vi "Initialize.vi"(7 "Baud Rate":u32(ring)=19200 items=["4800"=4800, "9600"=9600, "14400"=14400, "19200"=19200, "38400"=38400, "57600"=57600, "115200"=115200], 8 "error in (no error)":errorcluster, 9 "Reset (True)":bool=TRUE, 10 "ID Query (False)":bool, 11 "VISA resource name":refnum<visa-resource-name>) -> (0 "error out":errorcluster, 3 "VISA resource name out":refnum<visa-resource-name>)   [LabVIEW 2011, in "Ocean Server OS4000.lvlib"]
doc: "Establishes communication with the instrument and performs an instrument identification query. It also places the instrument in a default state needed for other instrument driver operations. Therefore, call this VI before calling other instrument driver VIs for this instrument. Generally, you need to call the Initialize VI only once at the beginning of an application."
uses:
  Ocean Server OS4000.lvlib
panel:
  # "(c) 2006 <National Instruments>.  ALL RIGHTS RESERVED."
  # "(c) 2009 National Instruments.  ALL RIGHTS RESERVED."
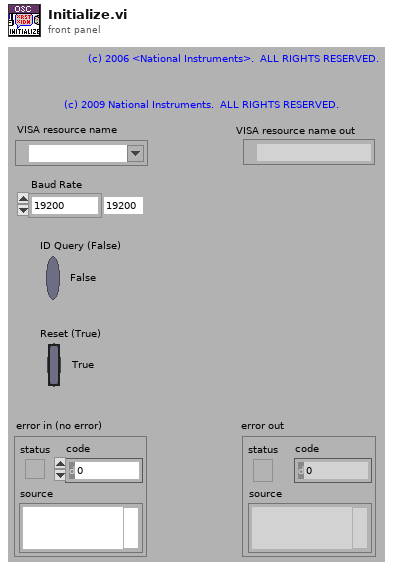
[diagram p1: front panel]
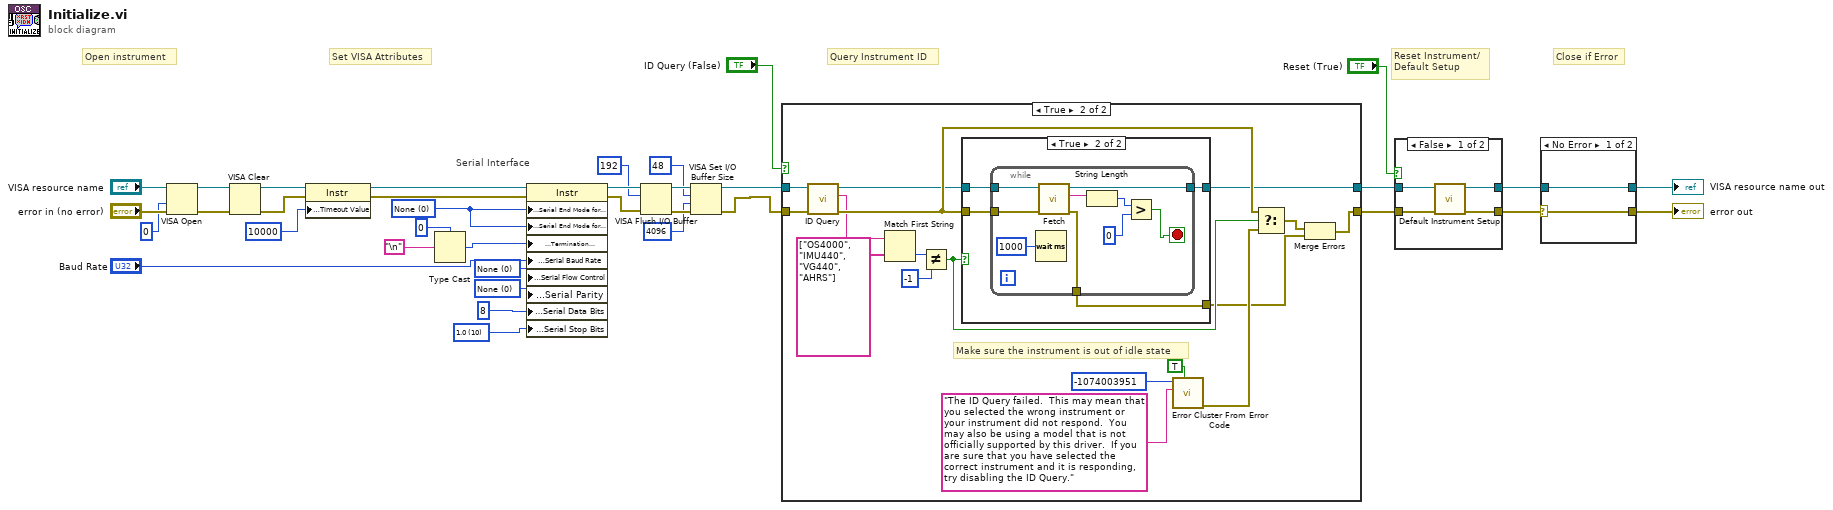
[diagram p0: block diagram]
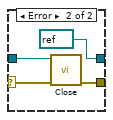
[diagram p2: hidden frame]
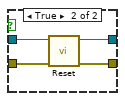
[diagram p3: hidden frame]
diagram:
  w1 = u16 10 items=["1.0"=10, "1.5"=15, "2.0"=20] ("Serial Settings:Stop Bits")
  w3 = u16 0 items=["None", "Odd", "Even", "Mark", "Space"] ("Serial Settings:Parity")
  w4 = u16 0 items=["None", "XON/XOFF", "RTS/CTS", "XON/XOFF & RTS/CTS", "DTR/DSR", "XON/XOFF & DTR/DSR"] ("Serial Settings:Flow Control")
  w8 = u16 0 items=["None", "LastBit", "TermChar"] ("Serial Settings:Serial End Mode for Reads")
  # "Serial Interface"
  # "Set VISA Attributes"
  # "Close if Error"
  # "Query Instrument ID"
  # "Reset Instrument/\nDefault Setup"
  # "Open instrument"
  n1 = VISA Open(access mode=u32 0, error in (no error)="error in (no error)", VISA resource name="VISA resource name") -> (VISA resource name=w24:refnum<visa-resource-name>, error out=w23:errorcluster)  [unwired: 2 in]
  n2 = VISA Clear(VISA resource name=w24, error in (no error)=w23) -> (VISA resource name out=w22:refnum<visa-resource-name>, error out=w21:errorcluster)
  n3 = property on="Property Node" class="Instr"(reference=w22, error in=w21, "General Settings:Timeout Value"=u32 10000) -> (reference out=w27:refnum<visa-resource-name>, error out=w26:errorcluster)
  n4 = Type Cast(type=0, x="\n" ("Line Feed Constant")) -> (*(type *) &x=w5:i32)
  n5 = property on="Property Node" class="Instr"(reference=w27, error in=w26, "Serial Settings:Serial End Mode for Reads"=w8, "Serial Settings:Serial End Mode for Writes"=w8, "Message Based Settings:Termination Character"=w5, "Serial Settings:Serial Baud Rate"="Baud Rate", "Serial Settings:Serial Flow Control"=w4, "Serial Settings:Serial Parity"=w3, "Serial Settings:Serial Data Bits"=u16 8 ("Serial Settings:Data Bits"), "Serial Settings:Serial Stop Bits"=w1) -> (reference out=w12:refnum<visa-resource-name>, error out=w14:errorcluster)
  n6 = VISA Flush I/O Buffer(VISA resource name=w12, mask (16)=u16 192, error in (no error)=w14) -> (VISA resource name out=w15:refnum<visa-resource-name>, error out=w13:errorcluster)
  n7 = VISA Set I/O Buffer Size(VISA resource name=w15, mask (16)=u16 48, size (4096)=u32 4096 ("size (0)"), error in (no error)=w13) -> (VISA resource name out=w29:refnum<visa-resource-name>, error out=w28:errorcluster)
  n8 = case shown="True" "ID Query (False)" {
    tunnel: [w37 w40] -> w35
    tunnel: [w38 w43] -> w36
    tunnel: w29 -> [w38 w51]
    tunnel: w28 -> [w37 w50]
    frame False {
    }
    frame True {
      # "Make sure the instrument is out of idle state"
      n9 = call "ID Query.vi"("error in (no error)"=w50, "VISA resource name"=w51) -> ("error out"=w45:errorcluster, "Model Name"=w39:string, "VISA resource name out"=w44:refnum<visa-resource-name>)  [unwired: 6 in, 1 out]
      n10 = Match First String(2:string[] ["OS4000", "IMU440", "VG440", "AHRS"], 3:w39) -> (0:w48:i32)  [unwired: 1 out]
      n11 = Not Equal?(x=w48, y=-1) -> (x != y?=w46:bool)
      n12 = case shown="True" w46 {
        tunnel: w44 -> [w57 w61]
        tunnel: w45 -> [w56 w60]
        tunnel: [w57 w59] -> w43
        tunnel: [w56 w58] -> w42
        frame False {
        }
        frame True {
          n13 = while {
            tunnel: w61 -> [w70]
            tunnel: w60 -> [w65]
            tunnel: [w64] -> w59
            tunnel: [w63] -> w58
            stop <- w66 stop-if-true
            n14 = Wait (ms)(milliseconds to wait=u32 1000) -> ()  [unwired: 1 out]
            n15 = call "Fetch.vi"("error in (no error)"=w65, "VISA resource name"=w70) -> ("error out"=w63:errorcluster, "Read Buffer"=w69:string, "VISA resource name out"=w64:refnum<visa-resource-name>)  [unwired: 5 in]
            n16 = String Length(string=w69) -> (length=w68:i32)
            n17 = Greater?(x=w68, y=0) -> (0:w66:bool)
          }
        }
      }
      n18 = call <vilib>:"Error Cluster From Error Code.vi"("show call chain? (False)"=TRUE, "error message (\"\")"="The ID Query failed.  This may mean that you selected the wrong instrument or your instrument did not respond.  You may also be using a model that is not officially supported by this driver.  If you are sure that you have selected the correct instrument and it is responding, try disabling the ID Query." ("Source (VI Name)"), "error code (0)"=-1074003951 ("Code")) -> ("error out"=w55:errorcluster)  [unwired: 6 in]
      n19 = Select(t=w45, s=w46, f=w55) -> (s? t:f=w41:errorcluster)
      n20 = Merge Errors(w41, w42) -> (w40:errorcluster)
    }
  }
  n21 = case shown="False" "Reset (True)" {
    tunnel: w35 -> [w73 w77]
    tunnel: [w71 w75] -> w17
    tunnel: w36 -> [w74 w78]
    tunnel: [w72 w76] -> w18
    frame False {
      n22 = call "Default Instrument Setup.vi"("error in (no error)"=w73, "VISA resource name"=w74) -> ("error out"=w71:errorcluster, "VISA resource out"=w72:refnum<visa-resource-name>)  [unwired: 8 in]
    }
    frame True {
      n23 = call "Reset.vi"("error in (no error)"=w77, "VISA resource name"=w78) -> ("error out"=w75:errorcluster, "VISA resource name out"=w76:refnum<visa-resource-name>)  [unwired: 8 in]
    }
  }
  n24 = case shown="No Error" w17 {
    selector: w17 -> [w79 w82]
    tunnel: w18 -> [w80 w83]
    tunnel: [w80 refnum<visa-resource-name> refnum ("VISA resource name out")] -> w20
    tunnel: [w79 w81] -> w19
    frame No Error {
    }
    frame Error {
      n25 = call "Close.vi"("error in (no error)"=w82, "VISA resource name"=w83) -> ("error out"=w81:errorcluster)  [unwired: 9 in]
    }
  }
  "VISA resource name out" <- w20
  "error out" <- w19
